vi "CspecCO2_2024.vi"(0 "Temperature [K]":dbl=293.15 format="%.4g") -> (1 "rel. unc Cp0/R CO2":dbl=0.0005 format="%.2e", 2 "Cp0/R CO2":dbl=4.440965545881931, 3 "Cp0 CO2 [J / Kmol]":dbl=36.9242419391239, 4 "Cv0 CO2 [J / Kmol]":dbl=28.609779339123904, 5 "Gamma0":dbl=1.2906161037261117)   [LabVIEW 2016]
panel:
  out "abs unc Cp0/R CO2":dbl=0.0011102413864704829 format="%#.4g"
  in  "rel. unc Cp0/R CO2":dbl=0.0005 format="%.2e"
  # "Based on spectroscopic calculations by Chao - validity between 10 K and 1500 K, as reported in Span & Wagner EoS for CO2 J. Phys. Chem. Ref. Data eq. 6.2 with coeffs in Table 27. Claimed to be accurate at 0.02 % level between 10 K and 1500 K with deviations from other calculations suppoting this claim. In contrast deviations from experimental data are larger, within 0.1%, likely because of exp. uncertainty. Conservatively we assume 0.05% rel. unc. \nThe prediction from a value reported by Zuckerwar at 273.15 K (see Table 16.7: Cp0/R=4.3233) is relatively different by 0.06 %. This value is coincident with Touloukian interpolation of 1970, with the coefficients reported by Zuckerwar (Table 3.1 vol. I)"
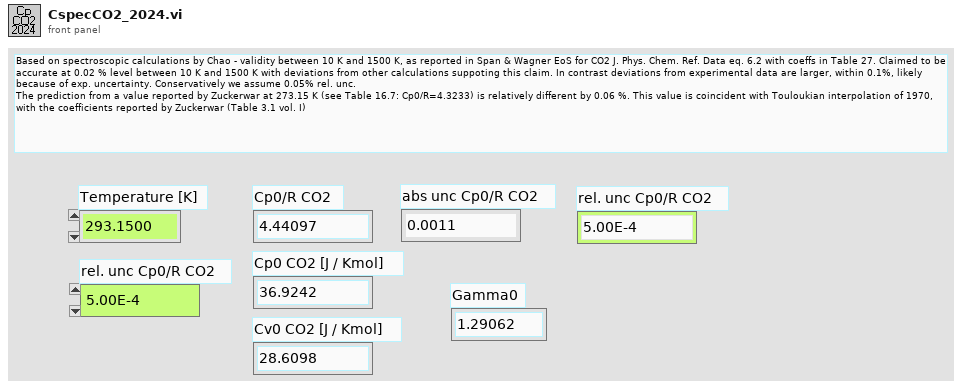
[diagram p1: front panel]
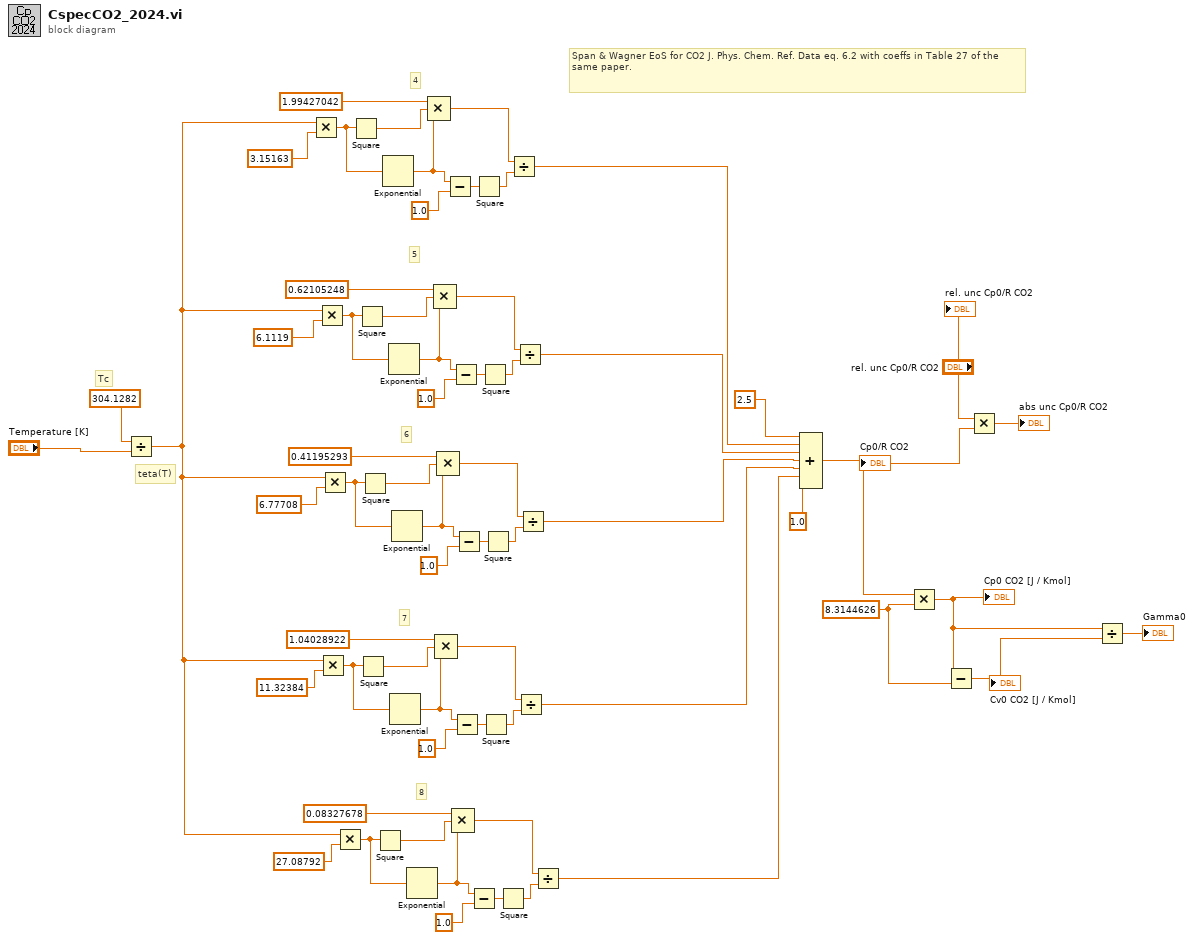
[diagram p0: block diagram]
diagram:
  w7 = 8.3144626
  # "Span & Wagner EoS for CO2 J. Phys. Chem. Ref. Data eq. 6.2 with coeffs in Table 27 of the same paper."
  # "Tc"
  # "8"
  # "7"
  # "4"
  # "6"
  # "5"
  # "teta(T)"
  n1 = Divide(x=304.1282, y="Temperature [K]") -> (x/y=w14:dbl)
  n2 = Multiply(x=w14, y=3.15163) -> (x*y=w57:dbl)
  n3 = Multiply(x=w14, y=6.1119) -> (x*y=w48:dbl)
  n4 = Multiply(x=w14, y=11.32384) -> (x*y=w29:dbl)
  n5 = Multiply(x=w14, y=6.77708) -> (x*y=w38:dbl)
  n6 = Multiply(x=w14, y=27.08792) -> (x*y=w20:dbl)
  n7 = Square(x=w57) -> (x^2=w59:dbl)
  n8 = Square(x=w48) -> (x^2=w50:dbl)
  n9 = Square(x=w29) -> (x^2=w31:dbl)
  n10 = Square(x=w38) -> (x^2=w40:dbl)
  n11 = Square(x=w20) -> (x^2=w22:dbl)
  n12 = Exponential(1:w57) -> (0:w55:dbl)
  n13 = Exponential(1:w48) -> (0:w46:dbl)
  n14 = Exponential(1:w29) -> (0:w27:dbl)
  n15 = Exponential(1:w38) -> (0:w36:dbl)
  n16 = Exponential(1:w20) -> (0:w18:dbl)
  n17 = Compound Arithmetic op=MULTIPLY(1.99427042, w59, w55) -> (w56:dbl)
  n18 = Compound Arithmetic op=MULTIPLY(0.62105248, w50, w46) -> (w47:dbl)
  n19 = Compound Arithmetic op=MULTIPLY(1.04028922, w31, w27) -> (w28:dbl)
  n20 = Compound Arithmetic op=MULTIPLY(0.41195293, w40, w36) -> (w37:dbl)
  n21 = Subtract(x=w55, y=1.0) -> (x-y=w53:dbl)
  n22 = Subtract(x=w46, y=1.0) -> (x-y=w44:dbl)
  n23 = Subtract(x=w27, y=1.0) -> (x-y=w25:dbl)
  n24 = Compound Arithmetic op=MULTIPLY(0.08327678, w22, w18) -> (w19:dbl)
  n25 = Subtract(x=w36, y=1.0) -> (x-y=w34:dbl)
  n26 = Subtract(x=w18, y=1.0) -> (x-y=w16:dbl)
  n27 = Square(x=w53) -> (x^2=w52:dbl)
  n28 = Square(x=w44) -> (x^2=w43:dbl)
  n29 = Square(x=w25) -> (x^2=w24:dbl)
  n30 = Square(x=w34) -> (x^2=w33:dbl)
  n31 = Square(x=w16) -> (x^2=w15:dbl)
  n32 = Divide(x=w56, y=w52) -> (x/y=w13:dbl)
  n33 = Divide(x=w47, y=w43) -> (x/y=w12:dbl)
  n34 = Divide(x=w28, y=w24) -> (x/y=w10:dbl)
  n35 = Divide(x=w37, y=w33) -> (x/y=w11:dbl)
  n36 = Divide(x=w19, y=w15) -> (x/y=w9:dbl)
  n37 = Compound Arithmetic op=ADD(2.5, w13, w12, w11, w10, w9, 1.0 ("value")) -> (w2:dbl)
  "Cp0/R CO2" <- w2
  n38 = Multiply(x=w2, y=w7) -> (x*y=w6:dbl)
  "Cp0 CO2 [J / Kmol]" <- w6
  n39 = Subtract(x=w6, y=w7) -> (x-y=w5:dbl)
  "Cv0 CO2 [J / Kmol]" <- w5
  n40 = Multiply(x="rel. unc Cp0/R CO2", y=w2) -> (x*y=→"abs unc Cp0/R CO2":dbl)
  n41 = Divide(x=w6, y=w5) -> (x/y=→"Gamma0":dbl)
  "rel. unc Cp0/R CO2" <- "rel. unc Cp0/R CO2"
